vi "Test Write Booleans.vi"(11 "TwinCAT ADS in":refnum<class "TwinCAT ADS.lvclass">) -> (3 "TwinCAT ADS out":refnum<class "TwinCAT ADS.lvclass">)   [LabVIEW 2018]
uses:
  TwinCAT ADS Class/TwinCAT ADS.lvclass
  4782b519-43e7-4b8e-bd72-e209be860882.vi
  e7a7b24b-aede-49d7-b369-bb451e1de87e.vi
  35134fdf-550d-4e68-bb51-d808b9e45170.vi
  5d41566e-774f-429d-b227-b1997554776b.vi
  TwinCAT ADS Class/VIs/Data/Read.vi
  <vilib>/addons/_JKI Toolkits/Caraya/classes/Assert/Assert True.vi
  <vilib>/addons/_JKI Toolkits/Caraya/classes/Assert/Assert False.vi
  <vilib>/addons/_JKI Toolkits/Caraya/classes/Assert/Assert.lvclass
  <vilib>/addons/_JKI Toolkits/Caraya/classes/Test/Test.lvclass
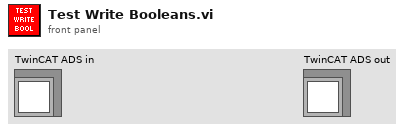
[diagram p1: front panel]
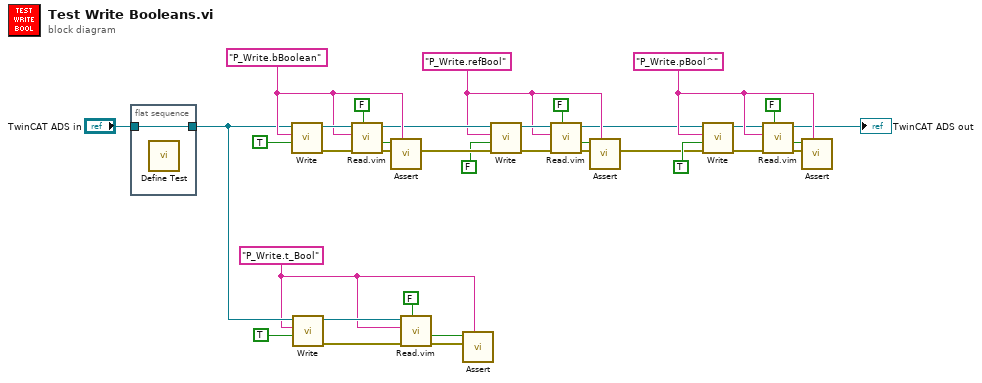
[diagram p0: block diagram]
diagram:
  w9 = "P_Write.pBool^" ("Symbol Name")
  w12 = "P_Write.refBool" ("Symbol Name")
  w26 = "P_Write.bBoolean" ("Symbol Name")
  w20 = "P_Write.t_Bool" ("Symbol Name")
  n1 = flat-sequence {
    tunnel: "TwinCAT ADS in" -> [w36]
    tunnel: [w36] -> w23
    frame #0 {
      n2 = call <vilib>:"Define Test.vi"() -> ()  [unwired: 10 in, 2 out]
    }
  }
  n3 = call "Write.vi"("Value"=TRUE, "Symbol Name"=w26, "TwinCAT ADS in"=w23) -> ("error out"=w25:errorcluster, "TwinCAT ADS out"=w35:refnum<class "TwinCAT ADS.lvclass">)  [unwired: 7 in]
  n4 = call "Write.vi"("Value"=TRUE, "Symbol Name"=w20, "TwinCAT ADS in"=w23) -> ("error out"=w21:errorcluster, "TwinCAT ADS out"=w22:refnum<class "TwinCAT ADS.lvclass">)  [unwired: 7 in]
  n5 = call "Read.vim"("Type"=FALSE, "error in (no error)"=w25, "Symbol Name"=w26, "TwinCAT ADS in"=w35) -> ("error out"=w33:errorcluster, "Value"=w32:bool, "TwinCAT ADS out"=w14:refnum<class "TwinCAT ADS.lvclass">)  [unwired: 5 in]
  n6 = call-poly <vilib>:"Assert.vi"("Label"=w26, "error in (no error)"=w33, "True?"=w32) -> ("error out"=w13:errorcluster)  [unwired: 7 in, 1 out]
  n7 = call "Read.vim"("Type"=FALSE, "error in (no error)"=w21, "Symbol Name"=w20, "TwinCAT ADS in"=w22) -> ("error out"=w29:errorcluster, "Value"=w30:bool)  [unwired: 5 in, 1 out]
  n8 = call-poly <vilib>:"Assert.vi"("Label"=w20, "error in (no error)"=w29, "True?"=w30) -> ()  [unwired: 7 in, 2 out]
  n9 = call "Write.vi"("error in (no error)"=w13, "Value"=FALSE, "Symbol Name"=w12, "TwinCAT ADS in"=w14) -> ("error out"=w19:errorcluster, "TwinCAT ADS out"=w15:refnum<class "TwinCAT ADS.lvclass">)  [unwired: 6 in]
  n10 = call "Read.vim"("Type"=FALSE, "error in (no error)"=w19, "Symbol Name"=w12, "TwinCAT ADS in"=w15) -> ("error out"=w17:errorcluster, "Value"=w18:bool, "TwinCAT ADS out"=w2:refnum<class "TwinCAT ADS.lvclass">)  [unwired: 5 in]
  n11 = call-poly <vilib>:"Assert.vi"("Label"=w12, "error in (no error)"=w17, "False?"=w18) -> ("error out"=w3:errorcluster)  [unwired: 7 in, 1 out]
  n12 = call "Write.vi"("error in (no error)"=w3, "Value"=TRUE, "Symbol Name"=w9, "TwinCAT ADS in"=w2) -> ("error out"=w4:errorcluster, "TwinCAT ADS out"=w8:refnum<class "TwinCAT ADS.lvclass">)  [unwired: 6 in]
  n13 = call "Read.vim"("Type"=FALSE, "error in (no error)"=w4, "Symbol Name"=w9, "TwinCAT ADS in"=w8) -> ("error out"=w6:errorcluster, "Value"=w5:bool, "TwinCAT ADS out"=→"TwinCAT ADS out":refnum<class "TwinCAT ADS.lvclass">)  [unwired: 5 in]
  n14 = call-poly <vilib>:"Assert.vi"("Label"=w9, "error in (no error)"=w6, "True?"=w5) -> ()  [unwired: 7 in, 2 out]
